vi "OpenGripper.vi"(8 "error in (no error)":errorcluster caption="Fehler (Eingang, kein Fehler)", 11 "Moveo Eingang":refnum<class "Moveo.lvclass">) -> (0 "error out":errorcluster caption="Fehler (Ausgang)", 3 "Moveo Ausgang":refnum<class "Moveo.lvclass">)   [LabVIEW 2019, in "Moveo.lvclass"]
uses:
  Moveo.lvclass
  Moveo.lvclass/Moveo.ctl
  MoveoSerialClass/MoveoSerial.lvclass
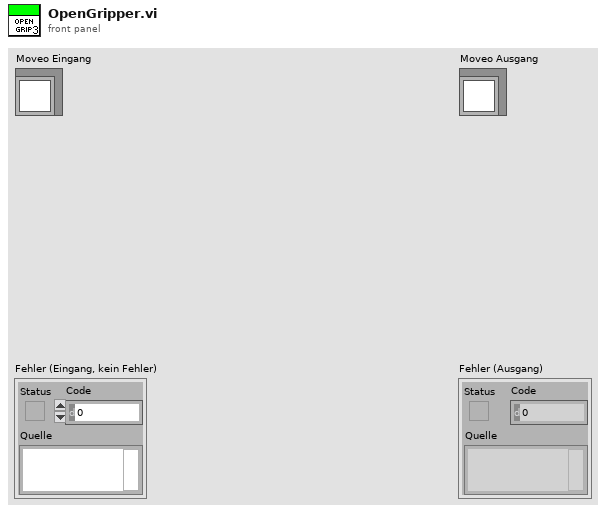
[diagram p1: front panel]
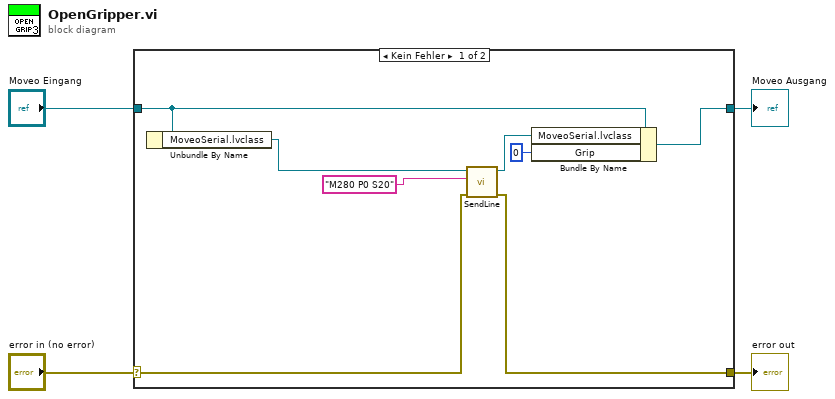
[diagram p0: block diagram]
diagram:
  n1 = case shown="Kein Fehler" "error in (no error)" {
    selector: "error in (no error)" -> [w7 w14]
    tunnel: [w6 w14] -> w3
    tunnel: [w9 w13] -> w1
    tunnel: "Moveo Eingang" -> [w10 w13]
    frame No Error {
      n2 = Unbundle By Name(w10) -> ("MoveoSerial.lvclass"=w11:refnum<class "MoveoSerial.lvclass">)
      n3 = call-dynamic "SendLine.vi"("error in (no error)"=w7, "SendString"="M280 P0 S20", "MoveoSerial Eingang"=w11) -> ("error out"=w6:errorcluster, "MoveoSerial Ausgang"=w8:refnum<class "MoveoSerial.lvclass">)  [unwired: 7 in]
      n4 = Bundle By Name(cluster=w10, "MoveoSerial.lvclass"=w8, "Grip"=i16 0) -> (w9:refnum<class "Moveo.lvclass">)
    }
    frame Error {
    }
  }
  "error out" <- w3
  "Moveo Ausgang" <- w1
